vi "Delete SN.vi"(8 "error in (no error)":errorcluster caption="entrée d'erreur (pas d'erreur)", 11 "Firebase Benches en entrée":refnum<class "Firebase Recovery_SN.lvclass">) -> (0 "error out":errorcluster caption="sortie d'erreur", 3 "Firebase Benches en sortie":refnum<class "Firebase Recovery_SN.lvclass">)   [LabVIEW 2020, in "Library Instrument & Equipement.lvlib" / "Library FireBase.lvlib" / "Firebase Recovery_SN.lvclass"]
doc: "Returns data according to Value_To_Find on Collection_to_find Use Nb_To_Read to determine the number to read\nPlease initialise the following values before use the VI\n - Name BDD\n - Value to find\n - API Key\n - Field Filter\n - Field Order\n - Collection_to_find\n\nIf there is no Field order -> Field Order=Field Filter"
uses:
  Firebase Recovery_SN.lvclass
  C:/Users/ngarcin/OneDrive - Altyor/Standard TB/Class/Firebase/Source/Firebase Driver/Firebase Driver.lvclass
  Firebase Recovery_SN.lvclass/Firebase Recovery_SN.ctl
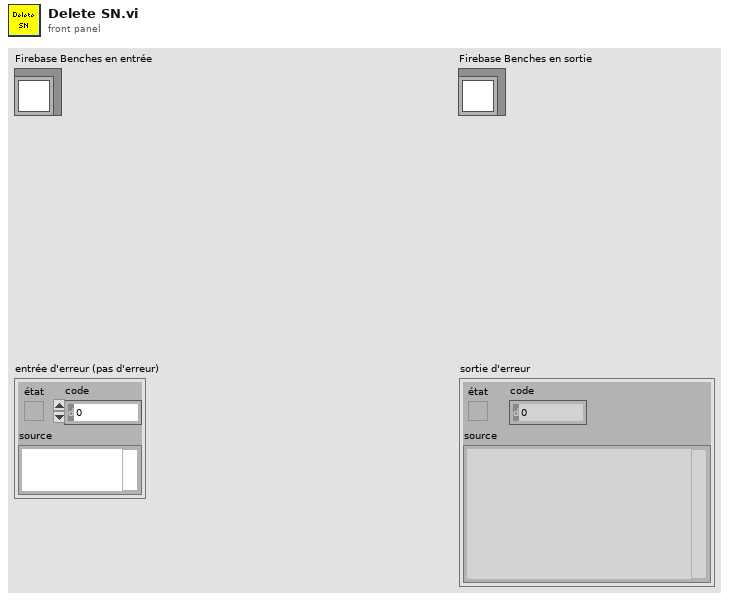
[diagram p1: front panel]
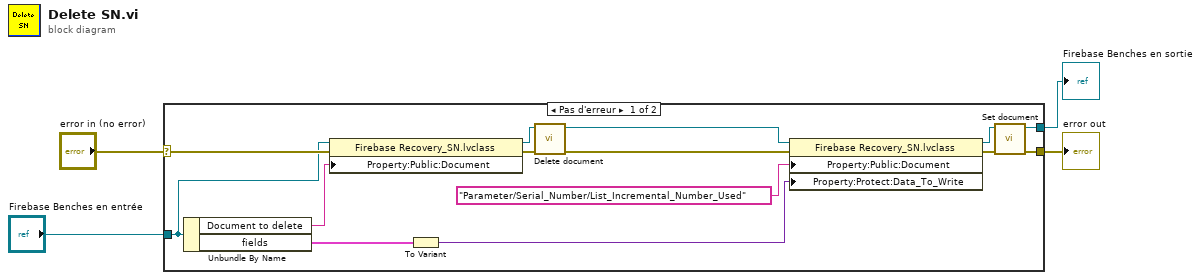
[diagram p0: block diagram]
diagram:
  n1 = case shown="Pas d'erreur" "error in (no error)" {
    selector: "error in (no error)" -> [w9 w20]
    tunnel: "Firebase Benches en entrée" -> [w7 w19]
    tunnel: [w10 w20] -> w3
    tunnel: [w11 w19] -> w2
    frame No Error {
      n2 = Unbundle By Name(w7) -> ("Document to delete"=w5:string, "fields"=w16:cluster{"Value":cluster{"stringValue":string}})
      n3 = property class="Firebase Recovery_SN.lvclass"(reference=w7, error in=w9, "Property:Public:Document"=w5) -> (reference out=w6:refnum<class "Firebase Recovery_SN.lvclass">, error out=w8:errorcluster)
      n4 = To Variant(anything=w16) -> (Variant=w15:variant)
      n5 = call-dynamic "Delete document.vi"("error in (no error)"=w8, "Firebase (Default) en entrée"=w6) -> ("error out"=w12:errorcluster, "Firebase (Default) en sortie"=w13:refnum<class "Firebase Recovery_SN.lvclass">)  [unwired: 8 in]
      n6 = property class="Firebase Recovery_SN.lvclass"(reference=w13, error in=w12, "Property:Public:Document"="Parameter/Serial_Number/List_Incremental_Number_Used" ("Collection_to_find"), "Property:Protect:Data_To_Write"=w15) -> (reference out=w17:refnum<class "Firebase Recovery_SN.lvclass">, error out=w18:errorcluster)
      n7 = call-dynamic "Set document.vi"("error in (no error)"=w18, "Firebase (Default) en entrée"=w17) -> ("error out"=w10:errorcluster, "Firebase (Default) en sortie"=w11:refnum<class "Firebase Recovery_SN.lvclass">)  [unwired: 8 in]
    }
    frame Error {
    }
  }
  "error out" <- w3
  "Firebase Benches en sortie" <- w2
